vi "GUI Tulip Tester.vi"() -> ()   [LabVIEW 2021]
panel:
  in  "Pass?":bool
  out "GUI Status":string
  out "GUI Table":string
  out "Ouset Table":string
  out "Ouset Status":string
  in  "ID Part":string
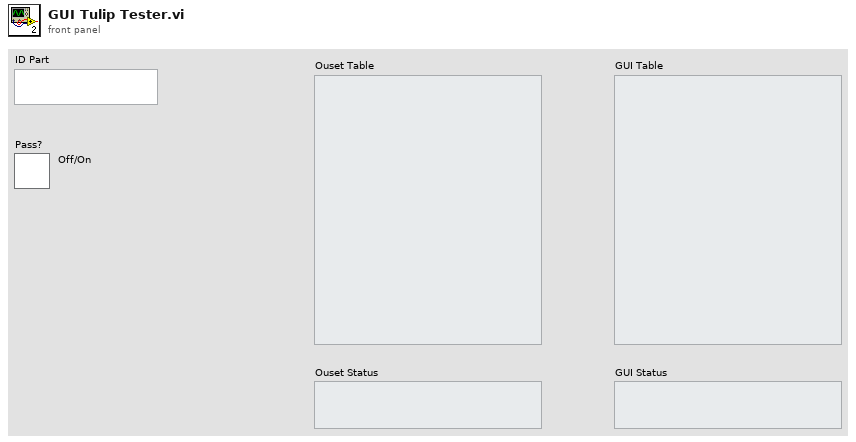
[diagram p1: front panel]
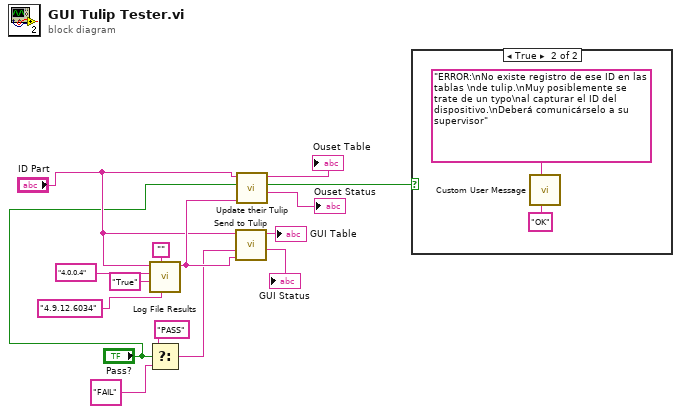
[diagram p0: block diagram]
diagram:
  n1 = call "Log File Results.vi"("Media version"="4.9.12.6034" ("OS build"), "Error"="", "Pass?"="True", "OS build"="4.0.0.4", "Part Number"="ID Part") -> ("File Name"=w13:string)  [unwired: 5 in, 1 out]
  n2 = Select(t="PASS", s="Pass?", f="FAIL") -> (s? t:f=w1:string)
  n3 = call "Send to Tulip.vi"("Data file"=w13, "Result"=w1, "Serial number"="ID Part") -> ("Status String"=→"GUI Status":string, "Response body"=→"GUI Table":string)  [unwired: 6 in, 1 out]
  n4 = call "Update their Tulip.vi"("Data file"=w13, "Test pass?"="Pass?", "Serial number"="ID Part") -> ("Status String"=→"Ouset Status":string, "Not Found?"=w12:bool, "Response body"=→"Ouset Table":string)  [unwired: 5 in, 1 out]
  n5 = case shown="True" w12 {
    frame False {
    }
    frame True {
      n6 = call "Custom User Message.vi"("Button text (\"OK\")"="OK" ("Button text (\"OK\")"), "MSG"="ERROR:\nNo existe registro de ese ID en las tablas \nde tulip.\nMuy posiblemente se trate de un typo\nal capturar el ID del dispositivo.\nDeberá comunicárselo a su supervisor" ("message")) -> ()  [unwired: 9 in, 1 out]
    }
  }
